vi "ADC Viewer.vi"() -> ()   [LabVIEW 2021]
doc: "This VI acts as an Adc Viewer where user gives the adc type specifications as inputs and can view the multiple channel data."
uses:
  Controls/Queue Operation.ctl
  Controls/State Cluster.ctl
  Controls/Adc Viewer Data.ctl
  Controls/ADC Type.ctl
  Classes/Model/Model.lvclass
  Controls/Channel U8 Array.ctl
  <vilib>/Waveform/DTblOps.llb/DTbl Append Digital Signals.vi
  <vilib>/Waveform/DWDTOps.llb/DWDT Append Digital Samples.vi
panel:
  in  "Help Button":bool
  out "Digital Waveform Graph":digitalwaveform[](graph)
  out "U8 data":u8[](array[numeric])
  out "Error Out":errorcluster
  in  "Error In":errorcluster
  in  "Channel Selection":string(tree)
  in  "ADC Type Specifications":T1={"Channels"="2", "Range"=180.0, "Resolution"=2.0, "Sampling Rate"=10.0} {"Sampling Rate" min=1.0 max=100.0; "Resolution" min=2.0 max=16.0; "Range" min=2.0 max=300.0}
  in  "Start/Stop":bool
  # "Analog to Digital Convertor Viewer"
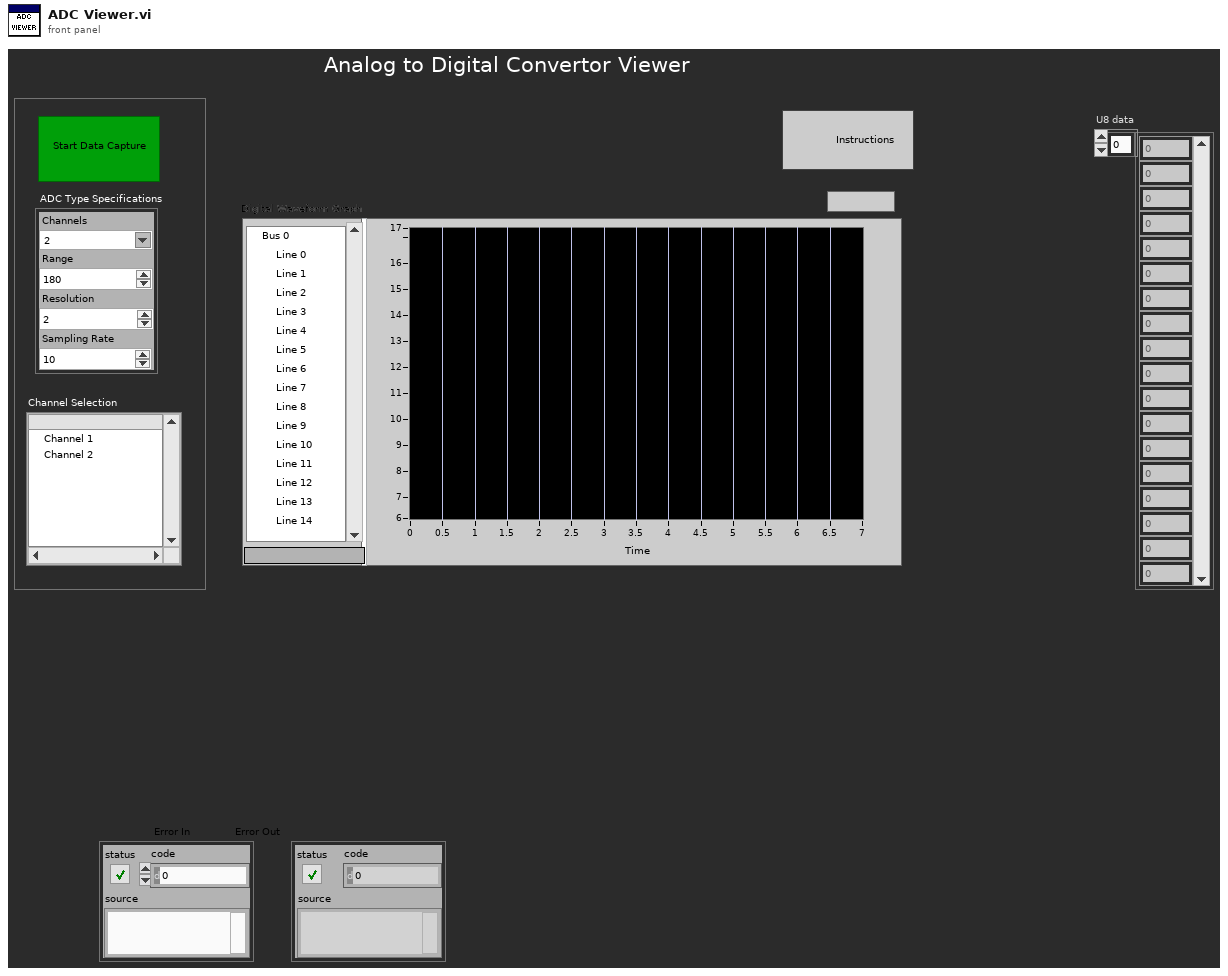
[diagram p1: front panel]
types:
  T1 = typedef "ADC Type.ctl" = cluster{"Channels":string, "Range":dbl, "Resolution":dbl, "Sampling Rate":dbl}
  T2 = typedef "State Cluster.ctl" = cluster{"State":string, "Data":variant}
  T3 = typedef "Queue Operation.ctl" = enum16{"Create", "Enqueue", "Enqueue N", "Enstack", "Dequeue", "Flush", "Release"}
  T4 = enum8{"Enabled", "Disabled", "Disabled and Grayed Out"}
  T5 = typedef "Adc Viewer Data.ctl" = cluster{"Start Time":dbl, "Stop User Event":refnum<user-event>, "Start/Stop":bool, "ADC Type":T1, "U8 Array":u8[], "reference out":refnum<vi>, "output waveform":digitalwaveform, "Digital array":digitalwaveform[], "analog waveform":waveform(dbl), "Model Class":refnum<class "Model.lvclass">, "Channel U8 Array":T6, "Selected Channel":string, "Display Array":u8[]}
  T6 = typedef "Channel U8 Array.ctl" = cluster{"Channel 1":u8[], "Channel 2":u8[], "Channel 3":u8[], "Channel 4":u8[]}
  T7 = typedef "LVPoint32TypeDef.ctl" = cluster{"Horizontal":i32, "Vertical":i32}
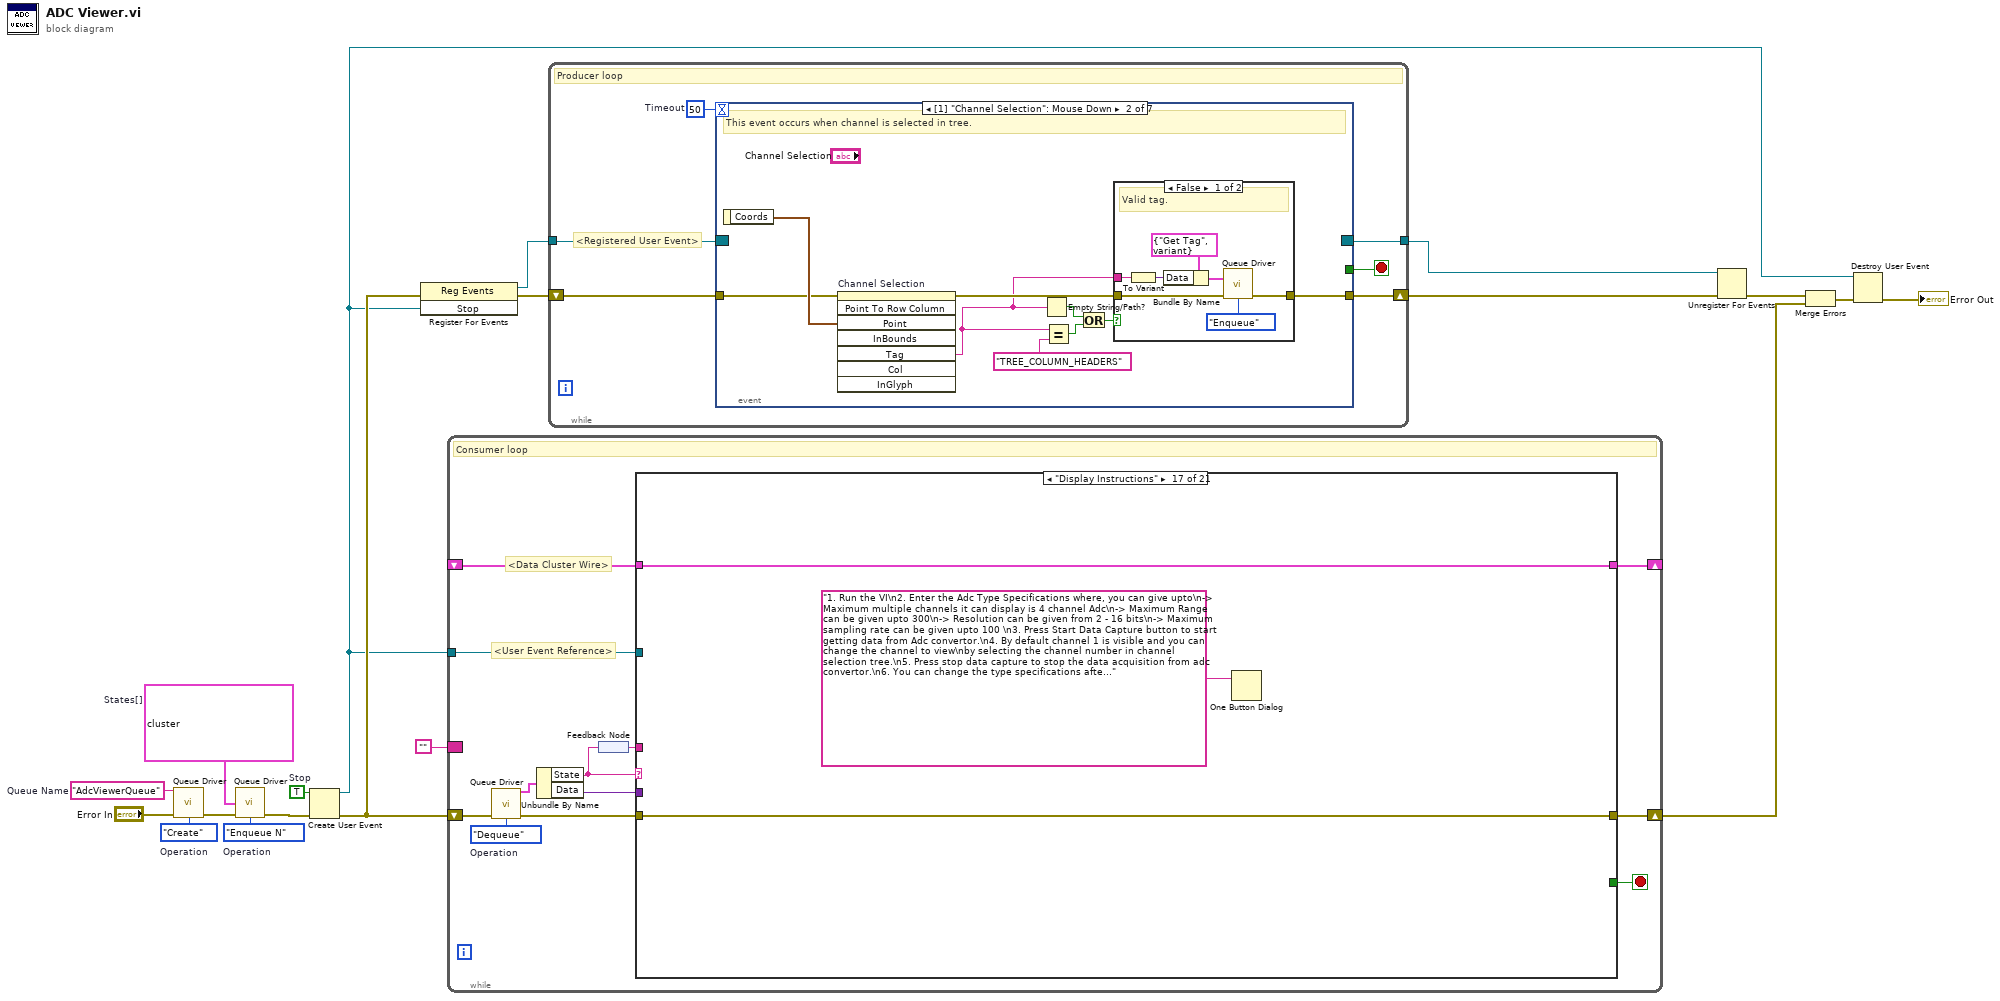
[diagram p0: block diagram]
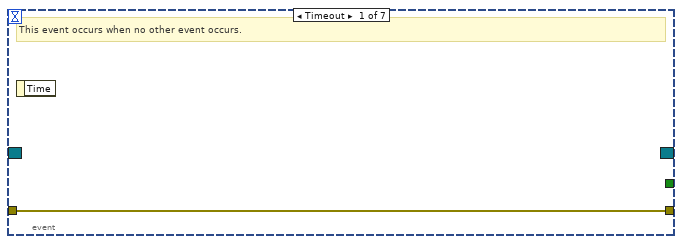
[diagram p2: hidden frame]
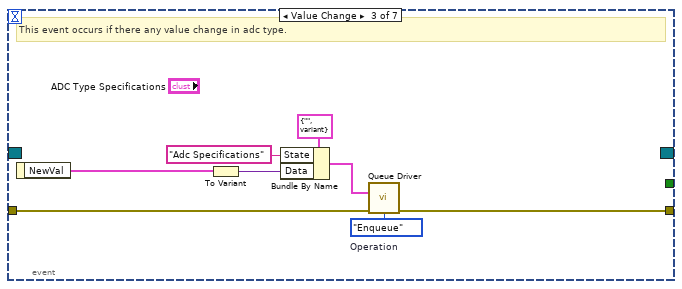
[diagram p4: hidden frame]
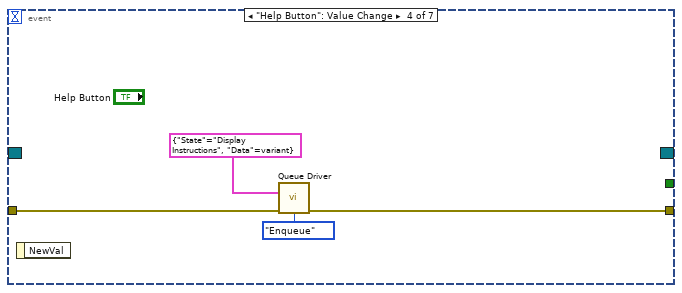
[diagram p5: hidden frame]
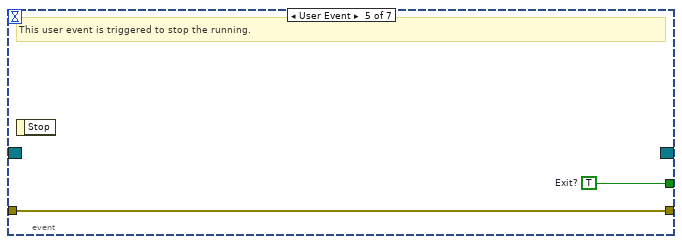
[diagram p6: hidden frame]
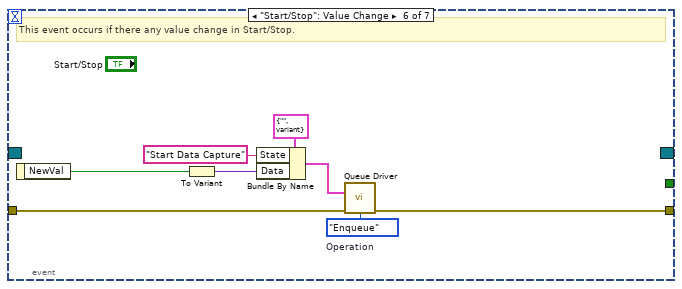
[diagram p7: hidden frame]
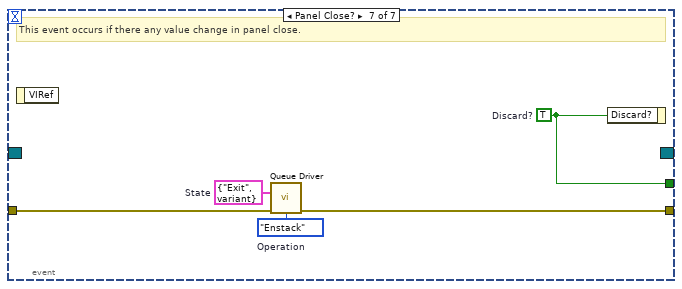
[diagram p8: hidden frame]
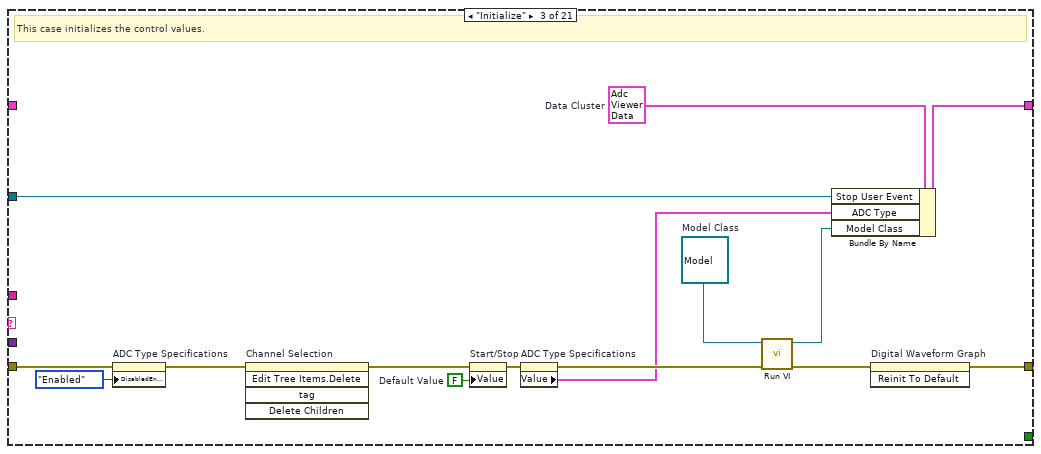
[diagram p11: hidden frame]
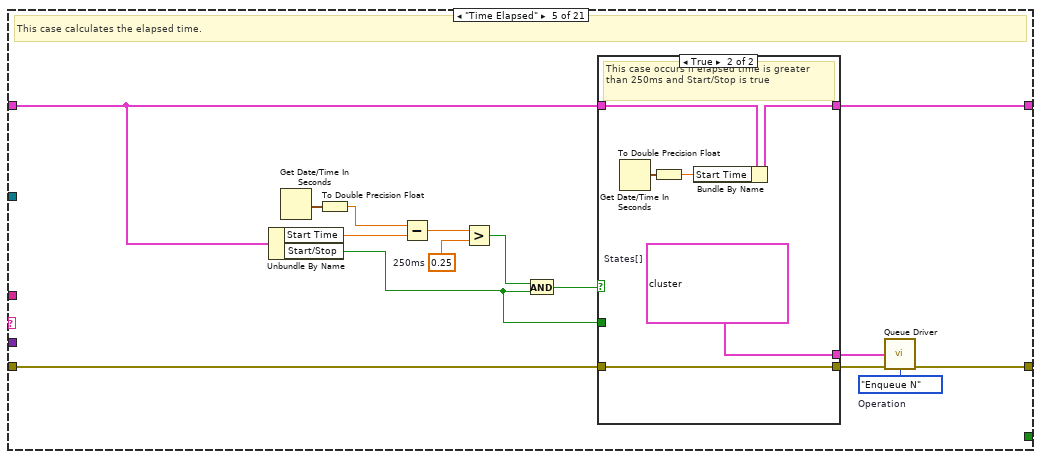
[diagram p13: hidden frame]
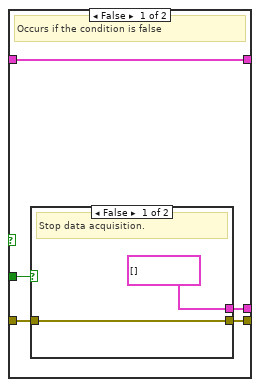
[diagram p14: hidden frame]
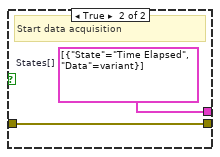
[diagram p15: hidden frame]
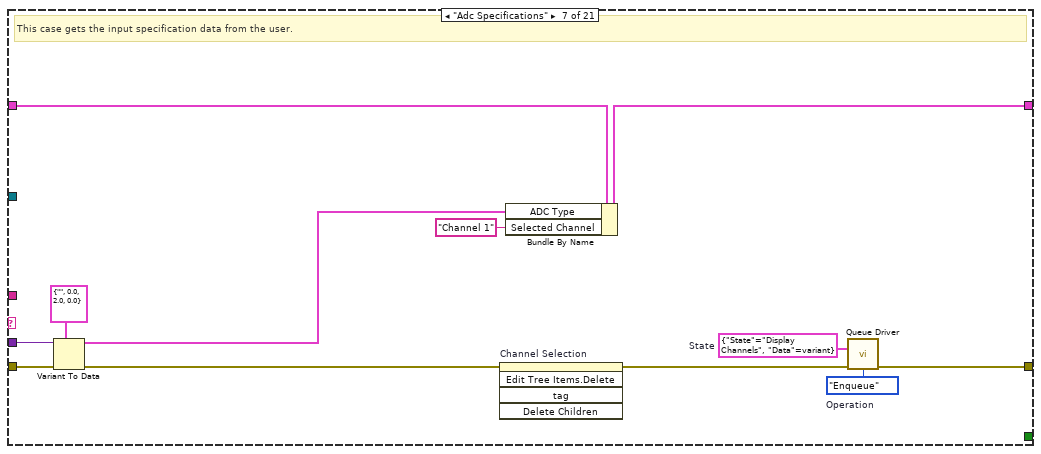
[diagram p17: hidden frame]
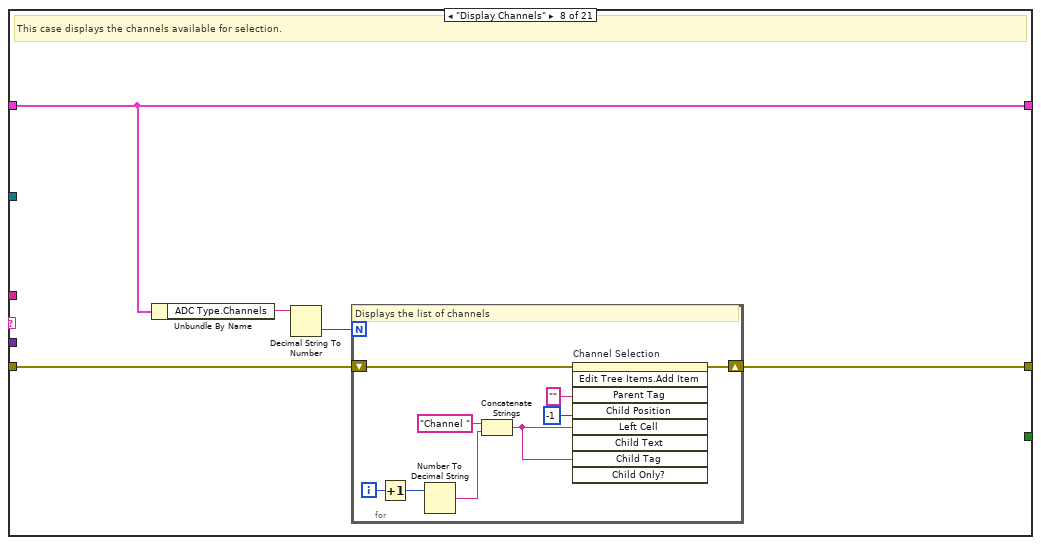
[diagram p18: hidden frame]
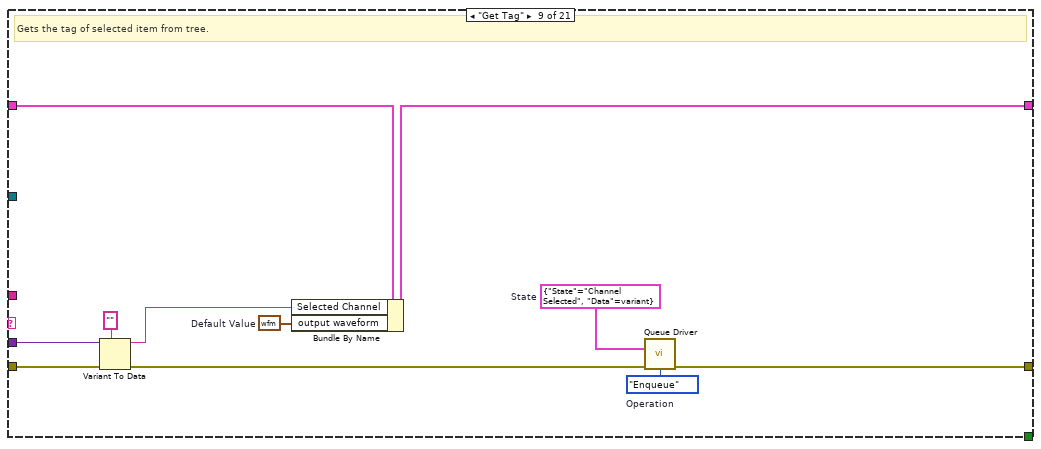
[diagram p19: hidden frame]
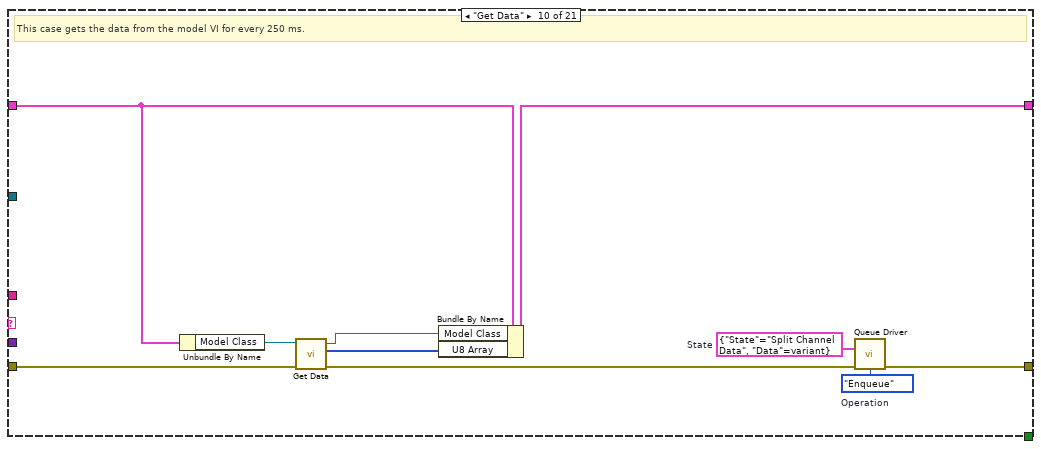
[diagram p20: hidden frame]
diagram:
  w7 = T2[] [{"State"="Initialize", "Data"=variant}, {"State"="Display Channels", "Data"=variant}]  # States[]
  w11 = TRUE  # Stop
  w15 = Queue_Operation."Enqueue N"  # Operation
  w17 = "AdcViewerQueue"  # Queue Name
  w18 = Queue_Operation."Create"  # Operation
  n1 = call "Queue Driver.vi"("Queue Name"=w17, "Error In"="Error In", "Operation"=w18) -> ("Error Out"=w16:errorcluster)  [unwired: 11 in, 1 out]
  n2 = call "Queue Driver.vi"("States[]"=w7, "Error In"=w16, "Operation"=w15) -> ("Error Out"=w12:errorcluster)  [unwired: 11 in, 1 out]
  n3 = Create User Event(user event datatype=w11, error in=w12) -> (user event=w2:refnum<user-event>, error out=w6:errorcluster)
  n4 = register-events(error in=w6, w2) -> (reference out=w9:refnum<event-registration>, error out=w10:errorcluster)  [unwired: 1 in]
  n5 = while {
    border: "" -> [_]
    shift-right: [w26] -> w8
    shift-left: w6 -> [w30]
    tunnel: w2 -> [w22]
    shift-right: [w24] -> _
    shift-left: _ -> [w25]
    stop <- w23 stop-if-true
    w31 = Queue_Operation."Dequeue"  # Operation
    # "<User Event Reference>"
    # "<Data Cluster Wire>"
    # "Consumer loop"
    n6 = call "Queue Driver.vi"("Error In"=w30, "Operation"=w31) -> ("Dequeued Element"=w29:T2, "Error Out"=w27:errorcluster)  [unwired: 12 in]
    n7 = Unbundle By Name(w29) -> ("State"=w21:string, "Data"=w20:variant)
    n8 = feedback-in #1(w21) -> ()
    n9 = feedback #1() -> (w28:string)
    n10 = case shown="\"Display Instructions\"" w21 {
      tunnel: w20 -> [_ _ _ _ _ _ w95 _ w120 _ w142 _ _ _ _ _ _ _ _ _ _]
      tunnel: w28 -> [_ _ _ _ _ _ _ _ _ _ _ _ _ _ _ _ _ _ w253 _ _]
      tunnel: w27 -> [w33 w35 w40 w52 w62 w84 w96 w99 w121 w125 w143 w182 w186 w216 w240 w244 w247 w249 w256 w274 w283]
      tunnel: [w33 w35 w36 w52 w58 w84 w90 w100 w113 w130 w138 w177 w185 w214 w240 w244 w247 w249 w252 w274 w277] -> w26
      tunnel: w25 -> [w32 w34 _ w51 w61 w83 w93 w101 w118 w127 w139 w180 w193 w218 w239 w243 w246 w248 w251 w273 w276]
      tunnel: [w32 w34 w50 w51 w60 w83 w92 w101 w117 w131 w140 w179 w187 w217 w239 w243 w246 w248 w251 w273 w276] -> w24
      tunnel: [_ _ _ _ _ _ _ _ _ _ _ _ _ _ _ _ _ _ _ _ w279] -> w23
      tunnel: w22 -> [_ _ w49 _ _ _ _ _ _ _ _ _ _ _ _ _ _ _ _ _ _]
      frame Default {
        # "This case occurs if there is any developer error."
      }
      frame "/**********  Initialize  ***********/" {
        # "Splitter case for initialization"
      }
      frame "Initialize" {
        w44 = T5 {"Start Time"=0.0, "Stop User Event"=refnum, "Start/Stop"=FALSE, "ADC Type"={"Channels"="", "Range"=0.0, "Resolution"=2.0, "Sampling Rate"=0.0}, "U8 Array"=[], "reference out"=refnum, "output waveform"={"t0"=timestamp(0 s since 1904-01-01), "dt"=0.0, "Y"={"transitions"=[], "data"=[]}}, "Digital array"=[], "analog waveform"={"t0"=timestamp(0 s since 1904-01-01), "dt"=1.0, "Y"=[]}, "Model Class"=refnum, "Channel U8 Array"={"Channel 1"=[], "Channel 2"=[], "Channel 3"=[], "Channel 4"=[]}, "Selected Channel"="", "Display Array"=[]}  # Data Cluster
        w46 = refnum<class "Model.lvclass"> refnum  # Model Class
        w48 = FALSE  # Default Value
        # "This case initializes the control values."
        n11 = property on="ADC Type Specifications" class="Clust (strict)"(error in=w40, "DisabledEnum"=T4."Enabled" ("Disabled")) -> (error out=w39:errorcluster)  [unwired: 1 in, 1 out]
        n12 = invoke on="Channel Selection" class="Tree (strict)" method="Edit Tree Items.Delete"(error in=w39) -> (error out=w47:errorcluster)  [unwired: 4 in, 4 out]
        n13 = property on="Start/Stop" class="Bool (strict)"(error in=w47, "Value"=w48) -> (error out=w43:errorcluster)  [unwired: 1 in, 1 out]
        n14 = property on="ADC Type Specifications" class="Clust (strict)"(error in=w43) -> (error out=w42:errorcluster, "Value"=w41:T1)  [unwired: 1 in, 1 out]
        n15 = call "Run VI.vi"("Error In"=w42, "Model In"=w46) -> ("Error Out"=w37:errorcluster, "Model out"=w45:refnum<class "Model.lvclass">)  [unwired: 8 in]
        n16 = Bundle By Name(cluster=w44, "Stop User Event"=w49, "ADC Type"=w41, "Model Class"=w45) -> (w50:T5)
        n17 = invoke on="Digital Waveform Graph" class="DigitalGraph (strict)" method="Reinit To Default"(error in=w37) -> (error out=w36:errorcluster)  [unwired: 2 in, 2 out]
      }
      frame "/********* Timer Functionalities **********/" {
        # "Splitter case for timer functionalities."
      }
      frame "Time Elapsed" {
        w57 = Queue_Operation."Enqueue N"  # Operation
        w63 = 0.25  # 250ms
        # "This case calculates the elapsed time."
        n18 = Unbundle By Name(w61) -> ("Start Time"=w65:dbl, "Start/Stop"=w53:bool)
        n19 = Get Date/Time In Seconds() -> (seconds since 1Jan1904=w67:timestamp)
        n20 = To Double Precision Float(number=w67) -> (double precision float=w66:dbl)
        n21 = Subtract(x=w66, y=w65) -> (x-y=w64:dbl)
        n22 = Greater?(x=w64, y=w63) -> (0:w55:bool)
        n23 = And(x=w55, y=w53) -> (x .and. y?=w54:bool)
        n24 = case shown="True" w54 {
          tunnel: w62 -> [w70 w77]
          tunnel: [w69 w77] -> w59
          tunnel: w61 -> [w72 w82]
          tunnel: [w72 w81] -> w60
          tunnel: [w71 w78] -> w56
          tunnel: w53 -> [w68 _]
          frame False {
            # "Occurs if the condition is false"
            n25 = case shown="False" w68 {
              tunnel: [T2[] [] ("States[]") w76] -> w71
              tunnel: [w74 w75] -> w69
              tunnel: w70 -> [w74 w75]
              frame False {
                # "Stop data acquisition."
              }
              frame True {
                w76 = T2[] [{"State"="Time Elapsed", "Data"=variant}]  # States[]
                # "Start data acquisition"
              }
            }
          }
          frame True {
            w78 = T2[] [{"State"="Get Data", "Data"=variant}, {"State"="Time Elapsed", "Data"=variant}]  # States[]
            # "This case occurs if elapsed time is greater than 250ms and Start/Stop is true"
            n26 = Get Date/Time In Seconds() -> (seconds since 1Jan1904=w79:timestamp)
            n27 = To Double Precision Float(number=w79) -> (double precision float=w80:dbl)
            n28 = Bundle By Name(cluster=w82, "Start Time"=w80) -> (w81:T5)
          }
        }
        n29 = call "Queue Driver.vi"("States[]"=w56, "Error In"=w59, "Operation"=w57) -> ("Error Out"=w58:errorcluster)  [unwired: 11 in, 1 out]
      }
      frame "/********  Functionalities *********/" {
        # "Splitter case for other functionalities."
      }
      frame "Adc Specifications" {
        w88 = T2 {"State"="Display Channels", "Data"=variant}  # State
        w89 = Queue_Operation."Enqueue"  # Operation
        # "This case gets the input specification data from the user."
        n30 = Variant To Data(error in=w96, type=T1 {"Channels"="", "Range"=0.0, "Resolution"=2.0, "Sampling Rate"=0.0} ("ADC Type"), Variant=w95) -> (data=w91:T1, error out=w87:errorcluster)
        n31 = invoke on="Channel Selection" class="Tree (strict)" method="Edit Tree Items.Delete"(error in=w87) -> (error out=w86:errorcluster)  [unwired: 4 in, 4 out]
        n32 = Bundle By Name(cluster=w93, "ADC Type"=w91, "Selected Channel"="Channel 1") -> (w92:T5)
        n33 = call "Queue Driver.vi"("State"=w88, "Error In"=w86, "Operation"=w89) -> ("Error Out"=w90:errorcluster)  [unwired: 11 in, 1 out]
      }
      frame "Display Channels" {
        # "This case displays the channels available for selection."
        n34 = Unbundle By Name(w101) -> ("ADC Type.Channels"=w98:string)
        n35 = Decimal String To Number(string=w98) -> (number=w97:i32)  [unwired: 2 in, 1 out]
        n36 = for {
          N: w97 -> [_]
          shift-right: [w110] -> w100
          shift-left: w99 -> [w109]
          i -> [w106]
          # "Displays the list of channels"
          n37 = Increment(x=w106) -> (x+1=w105:i32)
          n38 = Number To Decimal String(number=w105) -> (decimal integer string=w104:string)  [unwired: 1 in]
          n39 = Concatenate Strings("Channel " ("string"), w104) -> (w103:string)
          n40 = invoke on="Channel Selection" class="Tree (strict)" method="Edit Tree Items.Add Item"(error in=w109, "Parent Tag"="", "Child Position"=-1, "Left Cell"=w103, "Child Tag"=w103) -> (error out=w110:errorcluster)  [unwired: 4 in, 8 out]
        }
      }
      frame "Get Tag" {
        w111 = T2 {"State"="Channel Selected", "Data"=variant}  # State
        w112 = Queue_Operation."Enqueue"  # Operation
        w115 = digitalwaveform {"t0"=timestamp(0 s since 1904-01-01), "dt"=0.0, "Y"={"transitions"=[], "data"=[]}}  # Default Value
        # "Gets the tag of selected item from tree."
        n41 = Variant To Data(error in=w121, type="" ("State"), Variant=w120) -> (data=w116:string, error out=w114:errorcluster)
        n42 = Bundle By Name(cluster=w118, "Selected Channel"=w116, "output waveform"=w115) -> (w117:T5)
        n43 = call "Queue Driver.vi"("State"=w111, "Error In"=w114, "Operation"=w112) -> ("Error Out"=w113:errorcluster)  [unwired: 11 in, 1 out]
      }
      frame "Get Data" {
        w128 = T2 {"State"="Split Channel Data", "Data"=variant}  # State
        w129 = Queue_Operation."Enqueue"  # Operation
        # "This case gets the data from the model VI for every 250 ms."
        n44 = Unbundle By Name(w127) -> ("Model Class"=w126:refnum<class "Model.lvclass">)
        n45 = call "Get Data.vi"("Error In"=w125, "Model in"=w126) -> ("Error Out"=w124:errorcluster, "Digital Data"=w123:u8[], "Model out"=w122:refnum<class "Model.lvclass">)  [unwired: 7 in]
        n46 = Bundle By Name(cluster=w127, "Model Class"=w122, "U8 Array"=w123) -> (w131:T5)
        n47 = call "Queue Driver.vi"("State"=w128, "Error In"=w124, "Operation"=w129) -> ("Error Out"=w130:errorcluster)  [unwired: 11 in, 1 out]
      }
      frame "Start Data Capture" {
        # "This case gets the data when start/stop data capture is pressed."
        n48 = Variant To Data(error in=w143, type=TRUE, Variant=w142) -> (data=w134:bool, error out=w137:errorcluster)
        n49 = Unbundle By Name(w139) -> ("Model Class"=w135:refnum<class "Model.lvclass">, "ADC Type"=w132:T1)
        n50 = call "Start Data Capture.vi"("Error In"=w137, "ADC Type in"=w132, "Start/Stop in"=w134, "Model in"=w135) -> ("Error Out"=w136:errorcluster, "Model out"=w133:refnum<class "Model.lvclass">)  [unwired: 6 in]
        n51 = case shown="True" w134 {
          selector: w134 -> [w148 w155]
          tunnel: w136 -> [w146 w158]
          tunnel: [w145 w152] -> w138
          tunnel: w139 -> [w150 w162]
          tunnel: [w149 w159] -> w140
          tunnel: w133 -> [w147 w154]
          frame False {
            # "False if start data capture is false."
            n52 = Bundle By Name(cluster=w150, "Start/Stop"=w148, "Model Class"=w147) -> (w149:T5)
            n53 = property on="ADC Type Specifications" class="Clust (strict)"(error in=w146, "DisabledEnum"=T4."Enabled" ("Disabled")) -> (error out=w145:errorcluster)  [unwired: 1 in, 1 out]
          }
          frame True {
            w156 = T2 {"State"="Time Elapsed", "Data"=variant}  # State
            w157 = Queue_Operation."Enqueue"  # Operation
            # "True if start data capture is true."
            n54 = Get Date/Time In Seconds() -> (seconds since 1Jan1904=w160:timestamp)
            n55 = To Double Precision Float(number=w160) -> (double precision float=w161:dbl)
            n56 = Bundle By Name(cluster=w162, "Start/Stop"=w155, "Start Time"=w161, "Model Class"=w154) -> (w159:T5)
            n57 = call "Queue Driver.vi"("State"=w156, "Error In"=w158, "Operation"=w157) -> ("Error Out"=w153:errorcluster)  [unwired: 11 in, 1 out]
            n58 = property on="ADC Type Specifications" class="Clust (strict)"(error in=w153, "DisabledEnum"=T4."Disabled and Grayed Out" ("Disabled")) -> (error out=w152:errorcluster)  [unwired: 1 in, 1 out]
          }
        }
      }
      frame "Split Channel Data" {
        w175 = T2 {"State"="Channel Selected", "Data"=variant}  # State
        w176 = Queue_Operation."Enqueue"  # Operation
        # "Builds the array with the data received for each channel"
        # "Splits the channel data from the received U8 array based on the channel flags."
        n59 = Unbundle By Name(w180) -> ("Channel U8 Array.Channel 1"=w174:u8[], "Channel U8 Array.Channel 2"=w172:u8[], "Channel U8 Array.Channel 3"=w170:u8[], "Channel U8 Array.Channel 4"=w168:u8[], "U8 Array"=w181:u8[])
        n60 = call "Split Channel Data.vi"("Input Array"=w181, "Error In"=w182) -> ("Channel 1 Data"=w173:u8[], "Channel 2 Data"=w171:u8[], "Channel 3 Data"=w169:u8[], "Channel 4 Data"=w167:u8[], "Error Out"=w178:errorcluster)  [unwired: 9 in]
        n61 = Build Array (concatenate)(w172, w171) -> (w165:u8[])
        n62 = Build Array (concatenate)(w170, w169) -> (w164:u8[])
        n63 = Build Array (concatenate)(w174, w173) -> (w166:u8[])
        n64 = Build Array (concatenate)(w168, w167) -> (w163:u8[])
        n65 = Bundle By Name(cluster=w180, "Channel U8 Array.Channel 1"=w166, "Channel U8 Array.Channel 2"=w165, "Channel U8 Array.Channel 3"=w164, "Channel U8 Array.Channel 4"=w163) -> (w179:T5)
        n66 = call "Queue Driver.vi"("State"=w175, "Error In"=w178, "Operation"=w176) -> ("Error Out"=w177:errorcluster)  [unwired: 11 in, 1 out]
      }
      frame "Channel Selected" {
        w183 = T2 {"State"="Build Digital Waveform", "Data"=variant}  # State
        w184 = Queue_Operation."Enqueue"  # Operation
        # "Gets the U8 array of selected channel."
        n67 = Unbundle By Name(w193) -> ("Selected Channel"=w192:string, "Channel U8 Array.Channel 1"=w191:u8[], "Channel U8 Array.Channel 2"=w190:u8[], "Channel U8 Array.Channel 3"=w189:u8[], "Channel U8 Array.Channel 4"=w188:u8[])
        n68 = case shown="\"Channel 1\", Default" w192 {
          tunnel: w193 -> [w196 w199 w202 w205]
          tunnel: w191 -> [w195 _ _ _]
          tunnel: w190 -> [_ w198 _ _]
          tunnel: w189 -> [_ _ w201 _]
          tunnel: w188 -> [_ _ _ w204]
          tunnel: [w194 w197 w200 w203] -> w187
          frame "Channel 1", Default {
            n69 = Bundle By Name(cluster=w196, "Display Array"=w195) -> (w194:T5)
          }
          frame "Channel 2" {
            n70 = Bundle By Name(cluster=w199, "Display Array"=w198) -> (w197:T5)
          }
          frame "Channel 3" {
            n71 = Bundle By Name(cluster=w202, "Display Array"=w201) -> (w200:T5)
          }
          frame "Channel 4" {
            n72 = Bundle By Name(cluster=w205, "Display Array"=w204) -> (w203:T5)
          }
        }
        n73 = call "Queue Driver.vi"("State"=w183, "Error In"=w186, "Operation"=w184) -> ("Error Out"=w185:errorcluster)  [unwired: 11 in, 1 out]
      }
      frame "Build Digital Waveform" {
        w209 = T2 {"State"="FP Update", "Data"=variant}  # State
        w213 = Queue_Operation."Enqueue"  # Operation
        # "This case builds the digital waveform."
        n74 = Unbundle By Name(w218) -> ("output waveform"=w208:digitalwaveform, "Display Array"=w212:u8[])
        n75 = Decimate 1D Array(w212) -> (w211:u8[], w210:u8[])
        n76 = for {
          shift-right: [w222] -> w215
          shift-left: w216 -> [w223]
          tunnel: w211 -> [w237] mode=indexing
          tunnel: w210 -> [w238] mode=indexing
          shift-right: [w219] -> w207
          shift-left: w208 -> [w221]
          # "Builds the digital waveform."
          n77 = Number To Boolean Array(number=w237) -> (Boolean array=w233:bool[])
          n78 = Number To Boolean Array(number=w238) -> (Boolean array=w229:bool[])
          n79 = Boolean To (0,1)(Boolean=w233) -> (0, 1=w232:i16[])
          n80 = Boolean To (0,1)(Boolean=w229) -> (0, 1=w230:i16[])
          n81 = Reverse 1D Array(array=w232) -> (reversed array=w225:i16[])
          n82 = Reverse 1D Array(array=w230) -> (reversed array=w224:i16[])
          n83 = To Unsigned Byte Integer(number=w225) -> (unsigned 8bit integer=w231:u8[])
          n84 = To Unsigned Byte Integer(number=w224) -> (unsigned 8bit integer=w227:u8[])
          n85 = Build Array(w227) -> (w226:u8[][])
          n86 = Build Array(w231) -> (w228:u8[][])
          n87 = Bundle By Name("data"=w228) -> (w235:digitaldata)  [unwired: 1 in]
          n88 = Bundle By Name("data"=w226) -> (w236:digitaldata)  [unwired: 1 in]
          n89 = call-poly <vilib>:"Append Digital Signals.vi"("digital data (low bits)"=w236, "digital data (high bits)"=w235) -> ("digital data out"=w234:digitaldata)  [unwired: 8 in, 1 out]
          n90 = Bundle By Name("Y"=w234) -> (w220:digitalwaveform)  [unwired: 1 in]
          n91 = call-poly <vilib>:"Append Digital Samples.vi"("error in (no error)"=w223, "digital waveform B"=w220, "digital waveform A"=w221) -> ("error out"=w222:errorcluster, "digital waveform out"=w219:digitalwaveform)  [unwired: 7 in]
        }
        n92 = Build Array(w207) -> (w206:digitalwaveform[])
        n93 = Bundle By Name(cluster=w218, "Digital array"=w206) -> (w217:T5)
        n94 = call "Queue Driver.vi"("State"=w209, "Error In"=w215, "Operation"=w213) -> ("Error Out"=w214:errorcluster)  [unwired: 11 in, 1 out]
      }
      frame "/******* Front Panel Updates *******/" {
        # "Splitter case for front panel updates."
      }
      frame "FP Update" {
        # "This case updates the front panel indicators."
        n95 = Unbundle By Name(w243) -> ("U8 Array"=→"U8 data":u8[], "Digital array"=→"Digital Waveform Graph":digitalwaveform[])
      }
      frame "Display Instructions" {
        n96 = One Button Dialog(message="1. Run the VI\n2. Enter the Adc Type Specifications where, you can give upto\n-> Maximum multiple channels it can display is 4 channel Adc\n-> Maximum Range can be given upto 300\n-> Resolution can be given from 2 - 16 bits\n-> Maximum sampling rate can be given upto 100 \n3. Press Start Data Capture button to start getting data from Adc convertor.\n4. By default channel 1 is visible and you can change the channel to view\nby selecting the channel number in channel selection tree.\n5. Press stop data capture to stop the data acquisition from adc convertor.\n6. You can change the type specifications after clicking stop data capture \nand press start data capture to view the data again.") -> ()  [unwired: 1 in, 1 out]
      }
      frame "/******* Error Handling ********/" {
        # "Splitter case for error handling."
      }
      frame "Error" {
        # "This case handles error."
        n97 = Unbundle By Name(w256) -> ("code"=w255:i32, "source"=w254:string)
        n98 = call <vilib>:"Clear Errors.vi"("error in (no error)"=w256) -> ("error out"=w263:errorcluster)  [unwired: 5 in, 1 out]
        n99 = Format Into String(format string="Error occurred in state \"%s\"!!\nError Code: %d\nError Source: %s\n\nDo you wish to continue?", error in=w263, w253, w255, w254) -> (resulting string=w262:string, error out=w257:errorcluster)  [unwired: 1 in]
        n100 = Two Button Dialog(message=w262, 1:"Exit" ("F button name (\"Cancel\")"), 2:"Continue" ("T button name (\"OK\")")) -> (T button?=w259:bool)
        n101 = Unbundle By Name(w251) -> ("Stop User Event"=w250:refnum<user-event>)
        n102 = Not(x=w259) -> (.not. x?=w258:bool)
        n103 = case shown="True" w258 {
          tunnel: w257 -> [w265 w271]
          tunnel: [w265 w272] -> w252
          tunnel: w250 -> [_ w267]
          frame False {
            # "Continue."
          }
          frame True {
            # "Stops the running VI."
            n104 = Generate User Event(user event=w267, event data cluster=TRUE ("event data"), error in=w271) -> (error out=w268:errorcluster)  [unwired: 1 in, 1 out]
            n105 = call "Queue Driver.vi"("State"=T2 {"State"="Exit", "Data"=variant}, "Error In"=w268, "Operation"=Queue_Operation."Enstack") -> ("Error Out"=w272:errorcluster)  [unwired: 11 in, 1 out]
          }
        }
      }
      frame "/********** Exit Case ********/" {
        # "Splitter case for exiting."
      }
      frame "Exit" {
        w279 = TRUE  # Exit?
        w280 = Queue_Operation."Flush"  # Operation
        w281 = Queue_Operation."Release"  # Operation
        # "This case stops the running VI"
        n106 = call "Queue Driver.vi"("Error In"=w283, "Operation"=w280) -> ("Error Out"=w282:errorcluster)  [unwired: 12 in, 1 out]
        n107 = call "Queue Driver.vi"("Error In"=w282, "Operation"=w281) -> ("Error Out"=w278:errorcluster)  [unwired: 12 in, 1 out]
        n108 = Unbundle By Name(w276) -> ("Model Class"=w275:refnum<class "Model.lvclass">)
        n109 = call "Exit.vi"("Error In"=w278, "Model in"=w275) -> ("Error Out"=w277:errorcluster)  [unwired: 8 in, 1 out]
      }
    }
  }
  n110 = while {
    shift-right: [w287] -> w14
    shift-left: w10 -> [w288]
    tunnel: w9 -> [w286]
    tunnel: [w284] -> w4
    stop <- w285 stop-if-true
    w289 = 50  # Timeout
    # "<Registered User Event>"
    # "Producer loop"
    n111 = event shown="[1] \"Channel Selection\": Mouse Down" {
      selector: w286 -> [_ _ _ _ _ _ _]
      dyn-events: [_ _ _ _ _ _ _] -> w284
      timeout: w289 -> [_ _ _ _ _ _ _]
      tunnel: w288 -> [w290 w298 w310 w319 w321 w329 w334]
      tunnel: [w290 w293 w309 w318 w321 w328 w333] -> w287
      tunnel: [_ _ _ _ w320 _ w330] -> w285
      event Timeout {
        # "This event occurs when no other event occurs."
        n112 = event-data() -> ()  [unwired: 1 in, 1 out]
      }
      event "Channel Selection": Mouse Down {
        # "This event occurs when channel is selected in tree."
        n113 = event-data() -> ("Coords"=w299:T7)  [unwired: 1 in]
        n114 = invoke on="Channel Selection" class="Tree (strict)" method="Point To Row Column"(error in=w298, "Point"=w299) -> (error out=w292:errorcluster, "Tag"=w291:string)  [unwired: 6 in, 6 out]
        n115 = Empty String/Path?(string/path=w291) -> (empty?=w295:bool)
        n116 = Equal?(x=w291, y="TREE_COLUMN_HEADERS") -> (x = y?=w296:bool)
        n117 = Or(x=w295, y=w296) -> (x .or. y?=w294:bool)
        n118 = case shown="False" w294 {
          tunnel: [w304 w307] -> w293
          tunnel: w292 -> [w305 w307]
          tunnel: w291 -> [w301 _]
          frame False {
            # "Valid tag."
            n119 = To Variant(anything=w301) -> (Variant=w303:variant)
            n120 = Bundle By Name(cluster=T2 {"State"="Get Tag", "Data"=variant} ("State"), "Data"=w303) -> (w300:T2)
            n121 = call "Queue Driver.vi"("State"=w300, "Error In"=w305, "Operation"=Queue_Operation."Enqueue") -> ("Error Out"=w304:errorcluster)  [unwired: 11 in, 1 out]
          }
          frame True {
            # "Invalid tag."
          }
        }
      }
      event Value Change {
        w315 = Queue_Operation."Enqueue"  # Operation
        # "This event occurs if there any value change in adc type."
        n122 = event-data() -> ("NewVal"=w308:T1)  [unwired: 1 in]
        n123 = To Variant(anything=w308) -> (Variant=w312:variant)
        n124 = Bundle By Name(cluster=T2 {"State"="", "Data"=variant} ("State"), "State"="Adc Specifications", "Data"=w312) -> (w311:T2)
        n125 = call "Queue Driver.vi"("State"=w311, "Error In"=w310, "Operation"=w315) -> ("Error Out"=w309:errorcluster)  [unwired: 11 in, 1 out]
      }
      event "Help Button": Value Change {
        n126 = event-data() -> ()  [unwired: 1 in, 1 out]
        n127 = call "Queue Driver.vi"("State"=T2 {"State"="Display Instructions", "Data"=variant}, "Error In"=w319, "Operation"=Queue_Operation."Enqueue") -> ("Error Out"=w318:errorcluster)  [unwired: 11 in, 1 out]
      }
      event User Event {
        w320 = TRUE  # Exit?
        # "This user event is triggered to stop the running."
        n128 = event-data() -> ()  [unwired: 1 in, 1 out]
      }
      event "Start/Stop": Value Change {
        w327 = Queue_Operation."Enqueue"  # Operation
        # "This event occurs if there any value change in Start/Stop."
        n129 = event-data() -> ("NewVal"=w324:bool)  [unwired: 1 in]
        n130 = To Variant(anything=w324) -> (Variant=w323:variant)
        n131 = Bundle By Name(cluster=T2 {"State"="", "Data"=variant} ("State"), "State"="Start Data Capture", "Data"=w323) -> (w322:T2)
        n132 = call "Queue Driver.vi"("State"=w322, "Error In"=w329, "Operation"=w327) -> ("Error Out"=w328:errorcluster)  [unwired: 11 in, 1 out]
      }
      event Panel Close? {
        w330 = TRUE  # Discard?
        w331 = T2 {"State"="Exit", "Data"=variant}  # State
        w332 = Queue_Operation."Enstack"  # Operation
        # "This event occurs if there any value change in panel close."
        n133 = event-data() -> ()  [unwired: 1 in, 1 out]
        n134 = call "Queue Driver.vi"("State"=w331, "Error In"=w334, "Operation"=w332) -> ("Error Out"=w333:errorcluster)  [unwired: 11 in, 1 out]
        n135 = event-data("Discard?"=w330) -> ()  [unwired: 1 in, 1 out]
      }
    }
  }
  n136 = Unregister For Events(event registration refnum=w4, error in=w14) -> (error out=w5:errorcluster)
  n137 = Merge Errors(w5, w8) -> (w13:errorcluster)
  n138 = Destroy User Event(user event=w2, error in=w13) -> (error out=→"Error Out":errorcluster)
